vi "Write Actions.vi"(8 "error in (no error)":errorcluster, 10 "Actions":T1, 11 "EventsAbstract in":refnum<class "EventsAbstract.lvclass">) -> (0 "error out":errorcluster, 3 "EventsAbstract out":refnum<class "EventsAbstract.lvclass">)   [LabVIEW 2019, in "EventsAbstract.lvclass"]
uses:
  EventsAbstract.lvclass
  TypeDef/Event Actions.ctl
  Modules/ModuleAbstract/TypeDef/Module Actions.ctl
  <vilib>/ActorFramework/Message Enqueuer/Message Enqueuer.lvclass
  EventsAbstract.lvclass/EventsAbstract.ctl
  Modules/ModuleAbstract/ModuleAbstract.lvclass
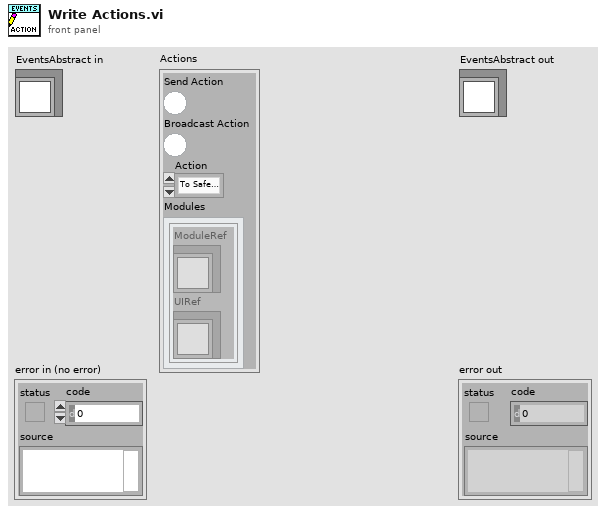
[diagram p1: front panel]
types:
  T1 = typedef "EventsAbstract.lvclass/Event Actions.ctl" = cluster{"Send Action":bool, "Broadcast Action":bool, "Action":T2, "Modules":cluster{"ModuleRef":refnum<class "Message Enqueuer.lvclass">, "UIRef":refnum<class "Message Enqueuer.lvclass">}[]}
  T2 = typedef "ModuleAbstract.lvlib/ModuleAbstract.lvclass/Module Actions.ctl" = enum16{"To Safe State", "Reset Safe State", "Close Module"}
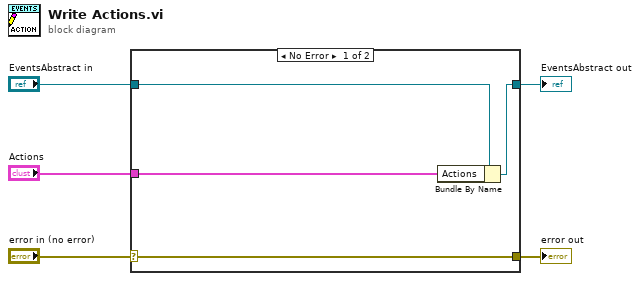
[diagram p0: block diagram]
diagram:
  n1 = case shown="No Error" "error in (no error)" {
    selector: "error in (no error)" -> [w9 w10]
    tunnel: [w9 w10] -> w4
    tunnel: [w7 w11] -> w2
    tunnel: "EventsAbstract in" -> [w8 w11]
    tunnel: "Actions" -> [w6 _]
    frame No Error {
      n2 = Bundle By Name(cluster=w8, "Actions"=w6) -> (w7:refnum<class "EventsAbstract.lvclass">)
    }
    frame Error {
    }
  }
  "error out" <- w4
  "EventsAbstract out" <- w2
